vi "Init Data.vi"(8 "error in (no error)":errorcluster, 10 "Data Object":refnum<class "Factory Plugin Framework.lvclass">, 11 "Skyworks - PVT in":refnum<class "Skyworks - PVT.lvclass">) -> (0 "error out":errorcluster, 3 "Skyworks - PVT out":refnum<class "Skyworks - PVT.lvclass">)   [LabVIEW 2018, in "Skyworks PVT.lvlib" / "Skyworks - PVT.lvclass"]
uses:
  Skyworks - PVT.lvclass
  C:/Sequence Automation/Plugins/Measurement Interface.lvlibp/Measurement Interface.lvclass
  Plugins/FPF.lvlibp/Factory Plugin Framework.lvclass
  Skyworks - PVT.lvclass/Skyworks - PVT.ctl
  Plugins/Measurement Interface.lvlibp/Private Methods/Measurement Parameters/Read Measurement Parameters.vi
  Plugins/Measurement Interface.lvlibp/Measurement Interface.lvclass
  Plugins/String Database.lvlibp/String Database.lvclass
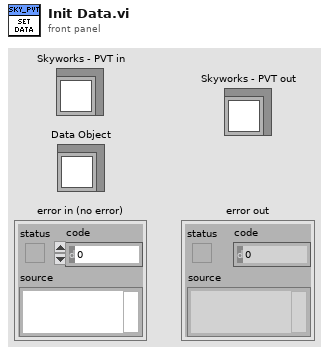
[diagram p1: front panel]
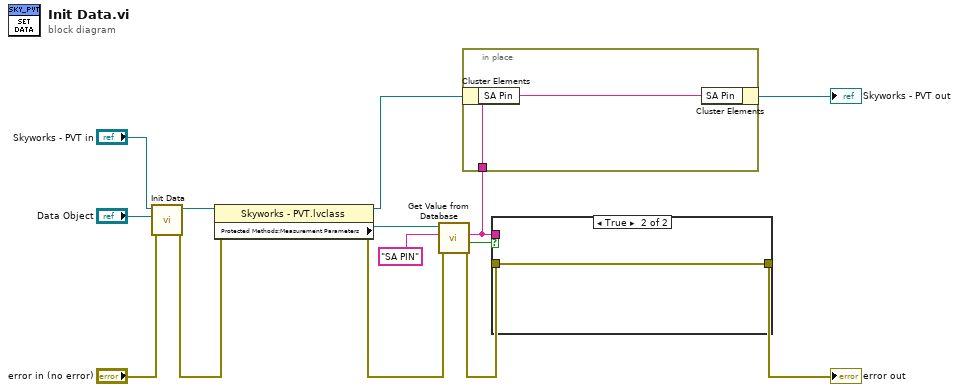
[diagram p0: block diagram]
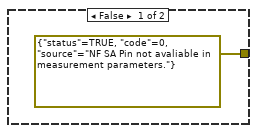
[diagram p2: hidden frame]
diagram:
  n1 = call-parent "Init Data.vi"("error in (no error)"="error in (no error)", "Data Object"="Data Object", "Measurement Interface in"="Skyworks - PVT in") -> ("error out"=w7:errorcluster, "Measurement Interface out"=w8:refnum<class "Skyworks - PVT.lvclass">)  [unwired: 7 in]
  n2 = property class="Skyworks - PVT.lvclass"(reference=w8, error in=w7) -> (reference out=w3:refnum<class "Skyworks - PVT.lvclass">, error out=w6:errorcluster, "Protected Methods:Measurement Parameters"=w11:refnum<class "String Database.lvclass">)
  n3 = call "Get Value from Database.vi"("error in (no error)"=w6, "Entry Name"="SA PIN", "Message in"=w11) -> ("error out"=w5:errorcluster, "Entry Found"=w9:bool, "Entry Value"=w2:string)  [unwired: 5 in, 1 out]
  n4 = in-place {
    in-place-border: w2 -> [w15]
    n5 = in-place-cluster #1(w3) -> ()  [unwired: 1 out]
    n6 = in-place-cluster #1("SA Pin"=w15) -> (→"Skyworks - PVT out":refnum<class "Skyworks - PVT.lvclass">)
  }
  n7 = case shown="True" w9 {
    tunnel: w5 -> [_ w17]
    tunnel: [errorcluster {"status"=TRUE, "code"=0, "source"="NF SA Pin not avaliable in measurement parameters."} ("error out") w17] -> w4
    tunnel: w2 -> [_ _]
    frame False {
    }
    frame True {
    }
  }
  "error out" <- w4
